vi "User Interface.vi"() -> ()   [LabVIEW 2015]
uses:
  <vilib>/Utility/error.llb/DialogType.ctl
  <vilib>/Instr/_visa.llb/VISA Configure Serial Port (Instr).vi
panel:
  out "Delta Psi 2":dbl
  out "Delta Psi":dbl
  out "Initial Stab":bool
  out "Initial Run":u32=1
  out "Automatic Mode Runtime":dbl
  out "ERROR":bool
  out "Theta i":dbl=177.58087201125176
  out "Psi i":dbl=181.08649789029536
  out "T initial read":u32
  out "Wzp":dbl(graph)
  out "Wyp":dbl(graph)=-0.09923664122137404
  out "Wxp":dbl(graph)=0.061068702290076333
  in  "Cluster":T1
  in  "Numeric":dbl=1.0
  out "return count":u32
  in  "Data Buffer":u8[](array[numeric])=[0, 8, 255, 243, 0, 0, 49, 1, 35, 1, 64, 0, 240, 0, 0, 3, 59, 255, 246, 0, 12, 0, 0, 48, 2, 35, 1, 64, 0, 240, 0, 0, 3, 27, 0, 0, 255, 244, 0, 0, 49, 1, 35, 1, 64, 0, 240, 0, 0, 2, 255, 0, 0, 255, 242, 0, 0, 49, 2, 35, 1, 64, 0, 240, 0, 0, 2, 225, 0, 9, 0, 0, 0, 0, 49, 1, 35, 1, 64, 0, 240, 0, 0, 2, 195, 0, 0, 0, 0, 0, 0, 48, 1, 35, 1, 64, 0, 240, 0, 0, 2, 167, 0, 0, 255, 248, 0, 0, 49, 1, 35, 1, 64, 0, 240, 0, 0, 2, 137, 0, 10, 0, 0, 0, 0, 49, 1, 35, 1, 64, 0, 240, 0, 0, 2, 109, 0, 0, 0, 0, 0, 0, 49, 1, 35, 1, 64, 0, 240, 0, 0, 2, 79, 0, 0, 0, 0, 0, 0, 49, 2, 35, 1, 64, 0, 240, 0, 0, 2, 49, 0, 0, 0, 0, 0, 0, 49, 1, 35, 1, 64, 0, 240, 0, 0, 2, 19, 0, 13, 255, 248, 0, 7, 49, 2, 35, 1, 64, 0, 240, 0, 0, 1, 247, 0, 0, 0, 12, 255, 245, 49, 1, 35, 1, 64, 0, 240, 0, 0, 1, 217, 0, 0, 0, 0, 0, 0, 49, 1, 35, 1, 64, 0, 240, 0, 0, 1, 189, 0, 0, 0, 12, 0, 0, 49, 1, 35, 1, 64, 0, 240, 0, 0, 1, 161, 0, 0, 255, 248, 0, 0, 49, 2, 35, 1, 64, 0, 240, 0, 0, 1, 131, 255, 249, 0, 0, 0, 9, 49, 2, 35, 1, 64, 0, 240, 0, 0, 1, 103, 0, 0, 255, 248, 0, 0, 49, 1, 35, 1, 64, 0, 240, 0, 0, 1, 74, 0, 0, 0, 0, 0, 0, 49, 1, 35, 1, 64, 0, 240, 0, 0, 1, 43, 0, 0, 0, 9, 0, 0, 49, 2, 35, 1, 64, 0, 240, 0, 0, 1, 13, 0, 0, 0, 7, 0, 0, 49, 2, 35, 1, 64, 0, 240, 0, 0, 0, 241, 0, 0, 0, 0, 0, 0, 49, 1, 35, 1, 64, 0, 240, 0, 0, 0, 211, 0, 0, 0, 0, 0, 0, 48, 2, 35, 1, 64, 0, 240, 0, 0, 0, 181, 0, 0, 0, 0, 0, 0, 49, 2, 35, 1, 64, 0, 240, 0, 0, 0, 151, 0, 0, 0, 0, 0, 0, 49, 1, 35, 1, 64, 0, 240, 0, 0, 0, 121, 0, 8, 0, 10, 0, 0, 48, 1, 35, 1, 64, 0, 240, 0, 0, 0, 91, 0, 0, 0, 0, 0, 0, 48, 2, 35, 1, 64, 0, 240, 0, 0, 0, 67, 0, 0, 0, 8, 0, 9, 48, 2, 35, 1, 64, 0, 240, 0, 0, 0, 63, 0, 0, 0, 0, 255, 243, 49, 2, 35, 1, 64, 0, 240, 0, 0, 0, 37, 0, 0, 0, 7, 0, 0, 49, 1, 35, 1, 64, 0, 240, 0, 0, 0, 5, 0, 0, 0, 0, 0, 0, 49, 2, 35, 1, 64, 0, 240, 0, 0, 0, 0]
  out "Psi":i16
  out "Theta":i16
  out "Cx":dbl=320.0
  out "Cy":dbl=240.0
  in  "Parity (0:none)":enum16{"None", "Odd", "Even", "Mark", "Space"}(ring)=enum."Even"
  in  "Phi B":dbl(slide) step=1.0 scale=-180.0..180.0
  in  "Psi B":dbl(slide) step=1.0 scale=-180.0..180.0
  in  "Theta B":dbl(slide) step=1.0 scale=-180.0..180.0
  in  "Tab Control":enum32{"MANUAL MODE", "AUTOMATIC MODE"}(tab)
  in  "Acquire \nTarget \nButton":bool
  in  "Yaw Angle":dbl(knob) caption="Pitch Angle" min=-90.0 max=90.0 step=1.0 scale=-90.0..90.0
  in  "Pitch Angle":dbl(knob) min=0.0 max=180.0 step=1.0
  in  "Start/Stop \nTracking":bool
  out "Target Position":dbl[][](graph)
  out "3D Picture":refnum<vi>(3d-picture)
  in  "stop":bool
  in  "VISA resource name":refnum<visa-resource-name>="COM4"
  in  "Stop bits (1 bit)":u16(ring)=10 items=["1.0"=10, "1.5"=15, "2.0"=20]
  in  "Baud rate":u32=115200
  # "SYSTEM SIMULATION"
  # "SERIAL COMMS SETUP"
  # "BASE MOTION"
  # "INERTIAL LOS RATES"
  # "SYSTEM STOP"
  # "SYSTEM COMMANDS"
  # "TARGET POSITION"
  # "Pitch Target"
  # "Yaw Target"
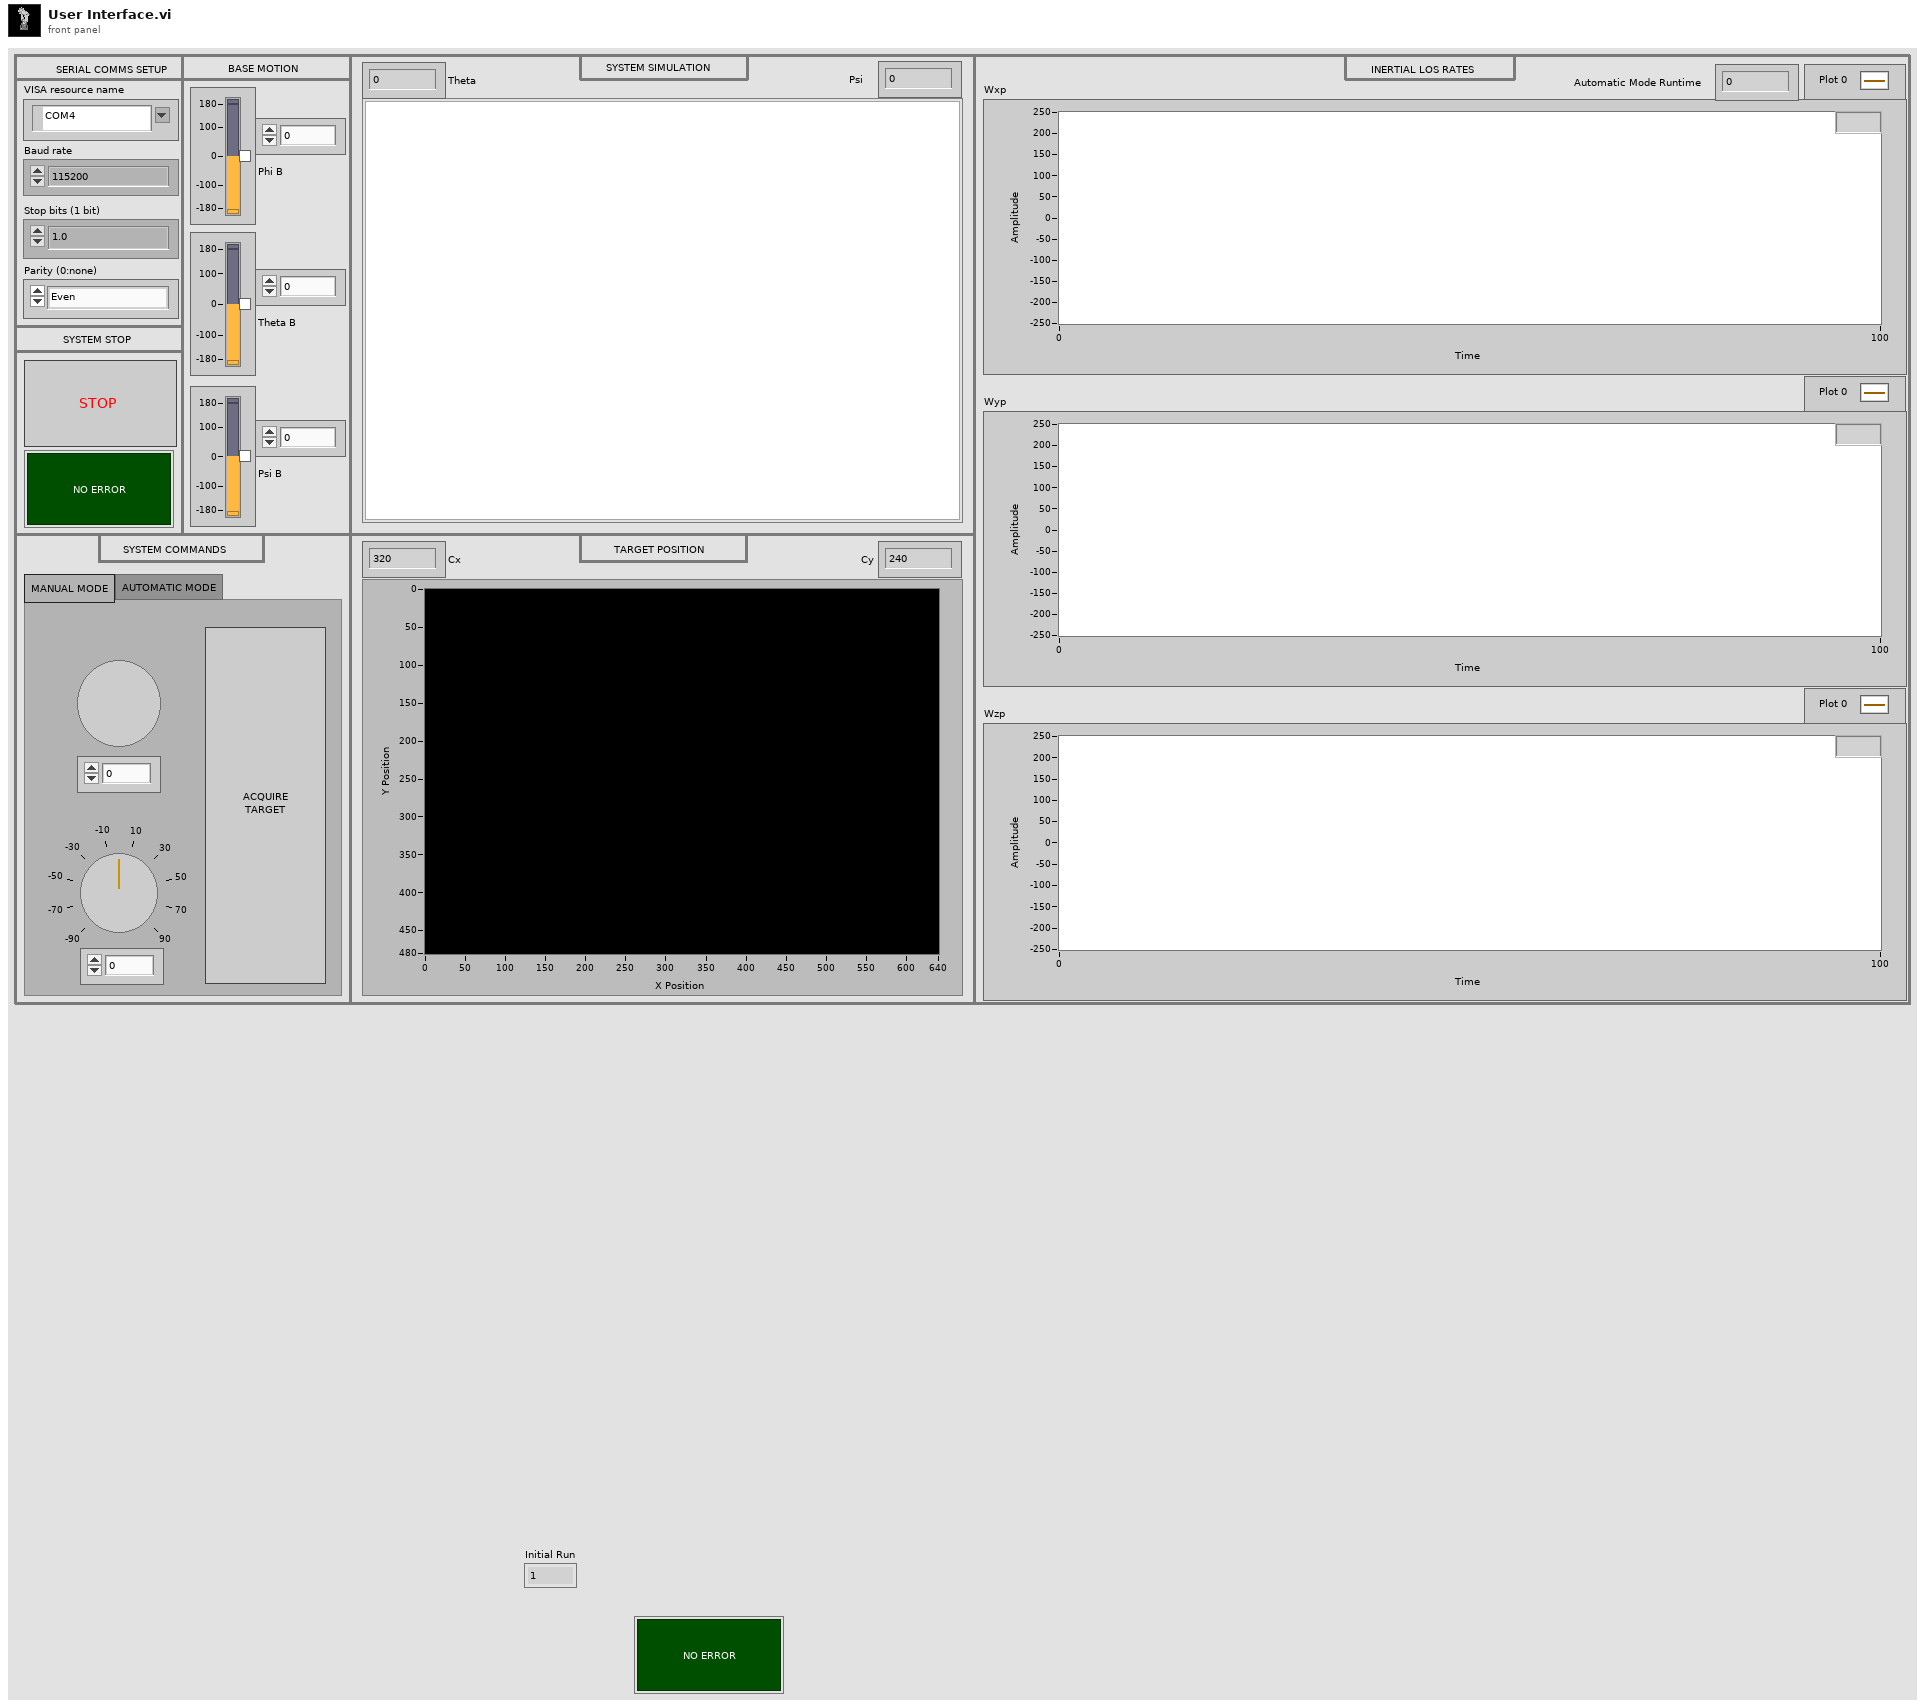
[diagram p1: front panel]
types:
  T1 = cluster{"X":dbl[], "Y":dbl[], "Z":dbl[], "theta":u16[], "phi":u16[], "CX":u16[], "CY":u16[], "Time":dbl[]}
  T2 = cluster{"Scene Object":refnum<vi>, "Base":refnum<vi>, "Gimbal":refnum<vi>, "Telescope":refnum<vi>, "error out":errorcluster}
  T3 = cluster{dbl[], dbl[], dbl[], u16[], u16[], u16[], u16[], dbl[]}
  T4 = typedef "DialogType.ctl" = u16
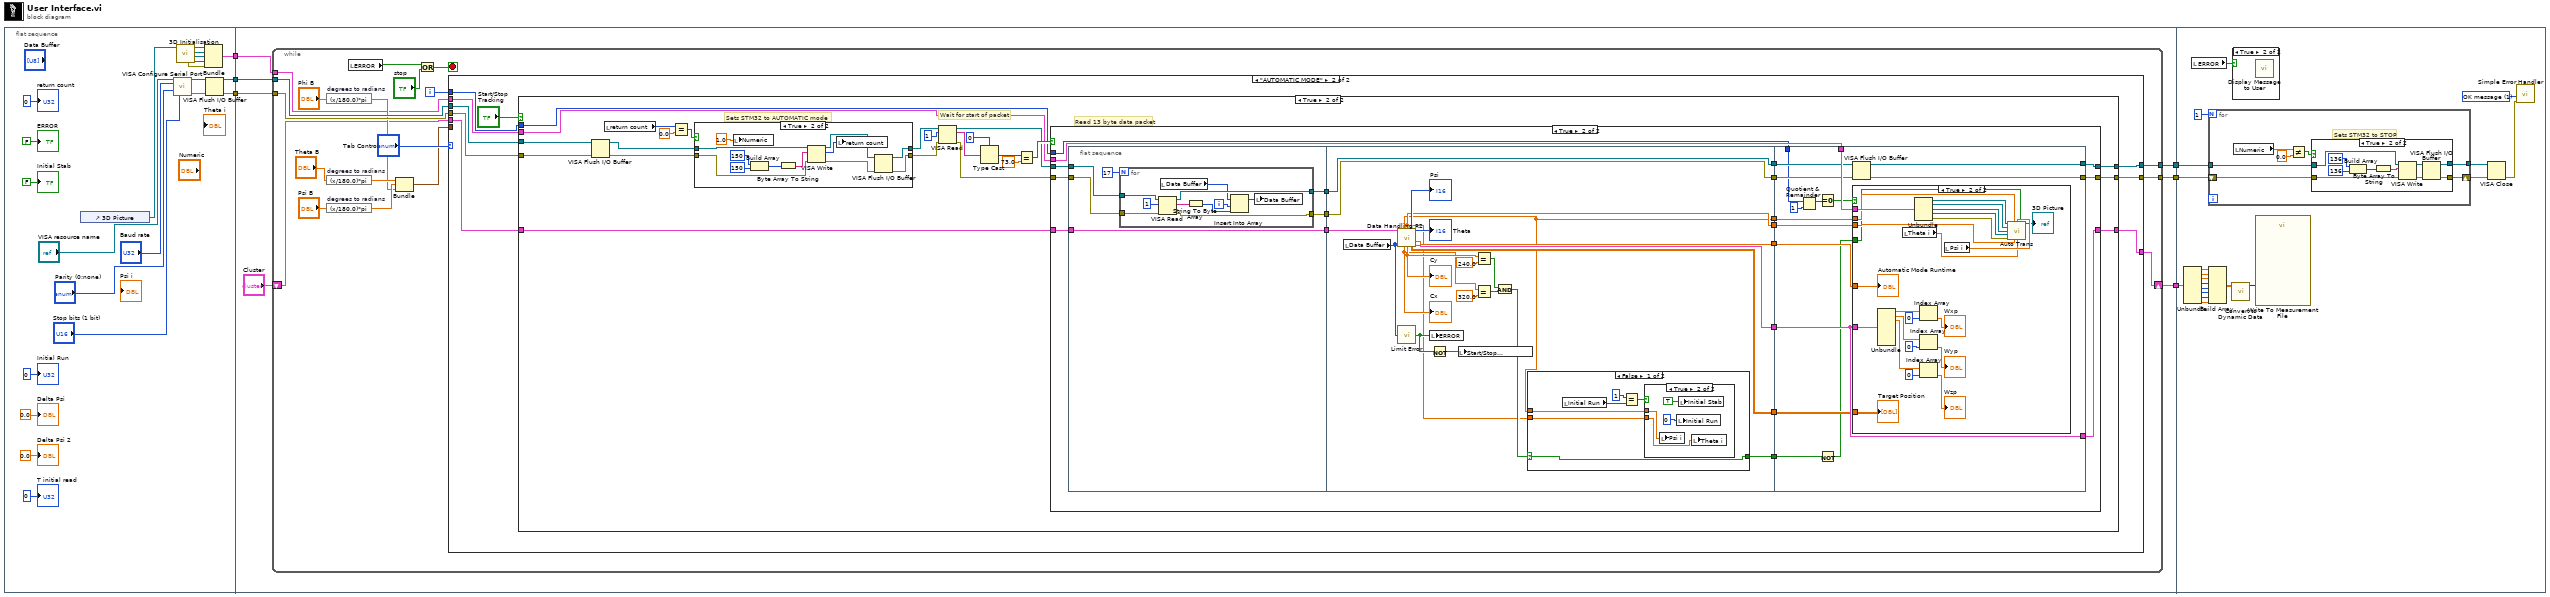
[diagram p0: block diagram]
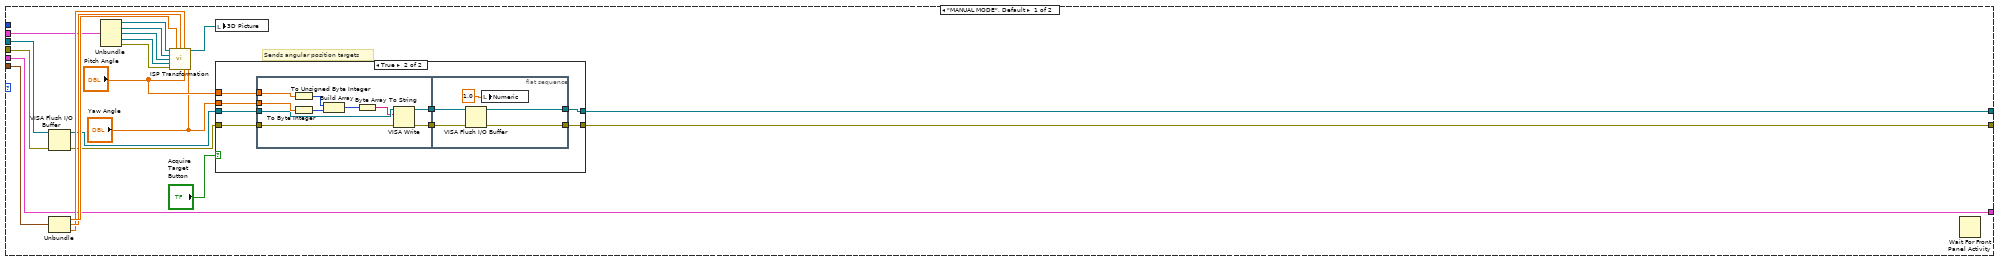
[diagram p2: hidden frame]
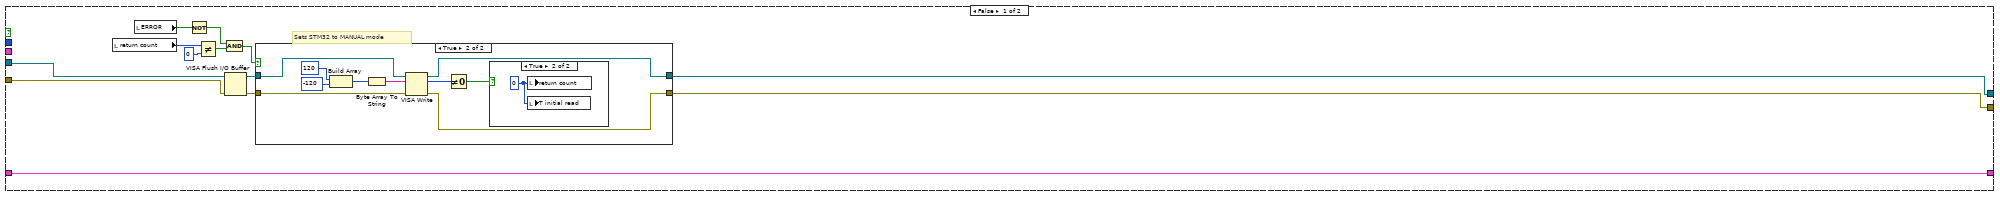
[diagram p4: hidden frame]
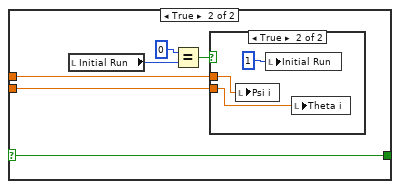
[diagram p9: hidden frame]
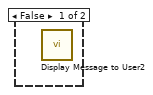
[diagram p14: hidden frame]
diagram:
  n1 = flat-sequence {
    tunnel: [w20] -> w6
    tunnel: [w19] -> w5
    tunnel: [w13] -> w4
    tunnel: w6 -> [w35]
    tunnel: w5 -> [w34]
    tunnel: w4 -> [w29]
    tunnel: [w32] -> w3
    tunnel: [w31] -> w2
    tunnel: [w30] -> w1
    tunnel: w3 -> [w308]
    tunnel: w2 -> [w307]
    tunnel: w1 -> [w306]
    frame #0 {
      n2 = control-ref of="3D Picture"() -> (w23:refnum<vi>)
      n3 = call-poly "VISA Configure Serial Port"("VISA resource name"="VISA resource name", "baud rate (9600)"="Baud rate", "parity (0:none)"="Parity (0:none)", "stop bits (10: 1 bit)"="Stop bits (1 bit)") -> ("VISA resource name out"=w22:refnum<visa-resource-name>, "error out"=w21:errorcluster)  [unwired: 10 in]
      n4 = call "3D Initialisation.vi"("reference"=w23) -> ("Telescope"=w15:refnum<vi>, "Gimbal"=w16:refnum<vi>, "Base"=w17:refnum<vi>, "Scene Object"=w18:refnum<vi>, "error out"=w14:errorcluster)  [unwired: 6 in]
      n5 = Bundle("Scene Object"=w18, "Base"=w17, "Gimbal"=w16, "Telescope"=w15, "error out"=w14) -> (w13:T2)  [unwired: 1 in]
      n6 = VISA Flush I/O Buffer(VISA resource name=w22, error in (no error)=w21) -> (VISA resource name out=w20:refnum<visa-resource-name>, error out=w19:errorcluster)  [unwired: 1 in]
      "return count" <- u32 0 ("return count")
      "T initial read" <- u32 0 ("initial read")
      "ERROR" <- FALSE ("LIMIT ERROR")
      "Initial Run" <- u32 0 ("initial read")
      "Initial Stab" <- FALSE ("LIMIT ERROR")
      "Delta Psi" <- 0.0 ("Delta Psi")
      "Delta Psi 2" <- 0.0 ("Delta Psi 2")
    }
    frame #1 {
      n7 = while {
        tunnel: w35 -> [w50]
        tunnel: w34 -> [w49]
        tunnel: w29 -> [w45]
        shift-right: [w43] -> w30
        shift-left: "Cluster" -> [w44]
        tunnel: [w42] -> w32
        tunnel: [w41] -> w31
        i -> [w36]
        stop <- w39 stop-if-true
        n8 = expression code="(x/180.0)*pi" "degrees to radians"("Phi B") -> (w46:dbl)
        n9 = expression code="(x/180.0)*pi" "degrees to radians"("Theta B") -> (w48:dbl)
        n10 = expression code="(x/180.0)*pi" "degrees to radians"("Psi B") -> (w47:dbl)
        n11 = local read "ERROR"() -> (w37:bool)
        n12 = Bundle("Theta B"=w48, "Psi B"=w47, "Phi B"=w46) -> (w40:cluster{"Theta B":dbl, "Psi B":dbl, "Phi B":dbl})  [unwired: 1 in]
        n13 = Or(x=w37, y="stop") -> (x .or. y?=w39:bool)
        n14 = case shown="\"AUTOMATIC MODE\"" "Tab Control" {
          tunnel: w50 -> [w56 w108]
          tunnel: w49 -> [w58 w107]
          tunnel: w44 -> [w63 w106]
          tunnel: w40 -> [w61 _]
          tunnel: w45 -> [w62 w105]
          tunnel: [w63 w104] -> w43
          tunnel: [w64 w103] -> w42
          tunnel: [w65 w102] -> w41
          tunnel: w36 -> [_ w101]
          frame "MANUAL MODE", Default {
            # "Sends angular position targets"
            n15 = VISA Flush I/O Buffer(VISA resource name=w56, error in (no error)=w58) -> (VISA resource name out=w55:refnum<visa-resource-name>, error out=w57:errorcluster)  [unwired: 1 in]
            n16 = Unbundle(w61) -> ("Theta B"=w70:dbl, "Psi B"=w69:dbl, "Phi B"=w68:dbl)
            n17 = Unbundle(w62) -> ("Scene Object"=w75:refnum<vi>, "Base"=w74:refnum<vi>, "Gimbal"=w73:refnum<vi>, "Telescope"=w72:refnum<vi>, "error out"=w71:errorcluster)
            n18 = call "ISP Transformation.vi"("Scene Object In"=w75, "Theta B"=w70, "Psi B"=w69, "Phi B"=w68, "Base"=w74, "Gimbal"=w73, "Telescope"=w72, "error in (no error)"=w71, "Theta"="Pitch Angle", "Psi"="Yaw Angle") -> ("Scene Object Out"=w67:refnum<vi>)  [unwired: 4 in, 1 out]
            n19 = local write "3D Picture"(w67) -> ()
            n20 = case shown="True" "Acquire \nTarget \nButton" {
              tunnel: "Pitch Angle" -> [_ w85]
              tunnel: "Yaw Angle" -> [_ w84]
              tunnel: w55 -> [w77 w83]
              tunnel: w57 -> [w76 w82]
              tunnel: [w76 w78] -> w65
              tunnel: [w77 w79] -> w64
              frame False {
              }
              frame True {
                n21 = flat-sequence {
                  tunnel: w85 -> [w95]
                  tunnel: w84 -> [w94]
                  tunnel: w83 -> [w93]
                  tunnel: w82 -> [w92]
                  tunnel: [w91] -> w81
                  tunnel: [w90] -> w80
                  tunnel: [w98] -> w78
                  tunnel: [w97] -> w79
                  tunnel: w81 -> [w96]
                  tunnel: w80 -> [w99]
                  frame #0 {
                    n22 = To Unsigned Byte Integer(number=w95) -> (unsigned 8bit integer=w87:u8)
                    n23 = To Byte Integer(number=w94) -> (8bit integer=w88:i8)
                    n24 = Build Array(w87, w88) -> (w89:u8[])
                    n25 = Byte Array To String(unsigned byte array=w89) -> (string=w86:string)
                    n26 = VISA Write(VISA resource name=w93, write buffer=w86, error in (no error)=w92) -> (VISA resource name out=w91:refnum<visa-resource-name>, error out=w90:errorcluster)  [unwired: 1 out]
                  }
                  frame #1 {
                    n27 = VISA Flush I/O Buffer(VISA resource name=w96, error in (no error)=w99) -> (VISA resource name out=w97:refnum<visa-resource-name>, error out=w98:errorcluster)  [unwired: 1 in]
                    n28 = local write "Numeric"(1.0 ("Numeric")) -> ()
                  }
                }
              }
            }
            n29 = Wait For Front Panel Activity() -> ()  [unwired: 3 in, 1 out]
          }
          frame "AUTOMATIC MODE" {
            n30 = case shown="True" "Start/Stop \nTracking" {
              tunnel: w108 -> [w113 w137]
              tunnel: w107 -> [w110 w136]
              tunnel: w106 -> [w118 w145]
              tunnel: w105 -> [_ w144]
              tunnel: [w118 w143] -> w104
              tunnel: [w120 w142] -> w103
              tunnel: [w119 w141] -> w102
              tunnel: w101 -> [_ w140]
              frame False {
                # "Sets STM32 to MANUAL mode"
                n31 = local read "return count"() -> (w121:u32)
                n32 = local read "ERROR"() -> (w115:bool)
                n33 = Not(x=w115) -> (.not. x?=w114:bool)
                n34 = Not Equal?(x=w121, y=u32 0) -> (x != y?=w116:bool)
                n35 = And(x=w114, y=w116) -> (x .and. y?=w117:bool)
                n36 = VISA Flush I/O Buffer(VISA resource name=w113, error in (no error)=w110) -> (VISA resource name out=w112:refnum<visa-resource-name>, error out=w111:errorcluster)  [unwired: 1 in]
                n37 = case shown="True" w117 {
                  tunnel: w112 -> [w124 w134]
                  tunnel: w111 -> [w123 w133]
                  tunnel: [w124 w132] -> w120
                  tunnel: [w123 w131] -> w119
                  frame False {
                  }
                  frame True {
                    n38 = Build Array(i8 120 ("element"), i8 -120 ("element")) -> (w127:i8[])
                    n39 = Byte Array To String(unsigned byte array=w127) -> (string=w130:string)
                    n40 = VISA Write(VISA resource name=w134, write buffer=w130, error in (no error)=w133) -> (VISA resource name out=w132:refnum<visa-resource-name>, return count=w125:u32, error out=w131:errorcluster)
                    n41 = Not Equal To 0?(x=w125) -> (x != 0?=w126:bool)
                    n42 = case shown="True" w126 {
                      frame False {
                      }
                      frame True {
                        w135 = u32 0 ("return count")
                        n43 = local write "return count"(w135) -> ()
                        n44 = local write "T initial read"(w135) -> ()
                      }
                    }
                  }
                }
              }
              frame True {
                # "Wait for start of packet"
                # "Read 13 byte data packet"
                # "Sets STM32 to AUTOMATIC mode"
                n45 = VISA Flush I/O Buffer(VISA resource name=w137, error in (no error)=w136) -> (VISA resource name out=w139:refnum<visa-resource-name>, error out=w138:errorcluster)  [unwired: 1 in]
                n46 = local read "return count"() -> (w156:u32)
                n47 = Equal?(x=w156, y=0.0) -> (x = y?=w158:bool)
                n48 = case shown="True" w158 {
                  tunnel: w139 -> [w278 w286]
                  tunnel: w138 -> [w277 w285]
                  tunnel: [w278 w281] -> w154
                  tunnel: [w277 w280] -> w153
                  frame False {
                  }
                  frame True {
                    n49 = local write "Numeric"(1.0 ("Numeric")) -> ()
                    n50 = Build Array(u8 150 ("element"), u8 150 ("element")) -> (w287:u8[])
                    n51 = Byte Array To String(unsigned byte array=w287) -> (string=w290:string)
                    n52 = VISA Write(VISA resource name=w286, write buffer=w290, error in (no error)=w285) -> (VISA resource name out=w284:refnum<visa-resource-name>, return count=w282:u32, error out=w283:errorcluster)
                    n53 = local write "return count"(w282) -> ()
                    n54 = VISA Flush I/O Buffer(VISA resource name=w284, error in (no error)=w283) -> (VISA resource name out=w281:refnum<visa-resource-name>, error out=w280:errorcluster)  [unwired: 1 in]
                  }
                }
                n55 = VISA Read(VISA resource name=w154, byte count=u32 1, error in (no error)=w153) -> (VISA resource name out=w147:refnum<visa-resource-name>, read buffer=w149:string, error out=w146:errorcluster)  [unwired: 1 out]
                n56 = Type Cast(type=u8 0, x=w149) -> (*(type *) &x=w151:u8)
                n57 = Equal?(x=w151, y=73.0) -> (x = y?=w148:bool)
                n58 = case shown="True" w148 {
                  tunnel: w147 -> [w160 w175]
                  tunnel: w146 -> [w159 w174]
                  tunnel: w145 -> [w161 w176]
                  tunnel: w144 -> [_ w180]
                  tunnel: [w161 w169] -> w143
                  tunnel: [w160 w179] -> w142
                  tunnel: [w159 w178] -> w141
                  tunnel: w140 -> [_ w177]
                  frame False {
                  }
                  frame True {
                    n59 = flat-sequence {
                      tunnel: w174 -> [w181]
                      tunnel: w175 -> [w182]
                      tunnel: [w185] -> w173
                      tunnel: [w184] -> w172
                      tunnel: w176 -> [w185]
                      tunnel: [w183] -> w171
                      tunnel: w173 -> [w207]
                      tunnel: w172 -> [w200]
                      tunnel: w171 -> [w201]
                      tunnel: [w201] -> w170
                      tunnel: [w206] -> w168
                      tunnel: [w205] -> w167
                      tunnel: [w204] -> w166
                      tunnel: [w203] -> w165
                      tunnel: [w202] -> w164
                      tunnel: [w200] -> w163
                      tunnel: [w199] -> w162
                      tunnel: [w243] -> w169
                      tunnel: w180 -> [w252]
                      tunnel: [w251] -> w179
                      tunnel: [w248] -> w178
                      tunnel: w177 -> [w247]
                      tunnel: w170 -> [w250]
                      tunnel: w168 -> [w243]
                      tunnel: w167 -> [w242]
                      tunnel: w166 -> [w241]
                      tunnel: w165 -> [w240]
                      tunnel: w164 -> [w239]
                      tunnel: w163 -> [w249]
                      tunnel: w162 -> [w238]
                      frame #0 {
                        n60 = for {
                          N: 17 -> [_]
                          tunnel: [w195] -> w183
                          tunnel: [w194] -> w184
                          tunnel: w182 -> [w188]
                          tunnel: w181 -> [w187]
                          i -> [w189]
                          n61 = VISA Read(VISA resource name=w188, byte count=u32 1, error in (no error)=w187) -> (VISA resource name out=w195:refnum<visa-resource-name>, read buffer=w193:string, error out=w194:errorcluster)  [unwired: 1 out]
                          n62 = local read "Data Buffer"() -> (w191:u8[])
                          n63 = String To Byte Array(string=w193) -> (unsigned byte array=w192:u8[])
                          n64 = Insert Into Array(array=w191, index=w189, new element=w192) -> (w190:u8[])
                          n65 = local write "Data Buffer"(w190) -> ()
                        }
                      }
                      frame #1 {
                        n66 = local read "Data Buffer"() -> (w208:u8[])
                        n67 = call "Data Handling R2.vi"("Cluster"=w207, "Data Buffer"=w208) -> ("Psi (image)"=w202:dbl, "Theta (image)"=w203:dbl, "Psi array out"=→"Psi":i16, "Theta array out"=→"Theta":i16, "Time"=w205:dbl, "Cx"=w213:dbl, "Cy"=w214:dbl, "Target array"=w204:dbl[][], "output cluster"=w206:T3)  [unwired: 5 in]
                        "Cy" <- w214
                        "Cx" <- w213
                        n68 = call "Limit Error.vi"("Array"=w208) -> ("LIMIT ERROR"=w210:bool)
                        n69 = local write "ERROR"(w210) -> ()
                        n70 = Not(x=w210) -> (.not. x?=w209:bool)
                        n71 = local write "Start/Stop \nTracking"(w209) -> ()
                        n72 = Equal?(x=w214, y=240.0) -> (x = y?=w198:bool)
                        n73 = Equal?(x=w213, y=320.0) -> (x = y?=w197:bool)
                        n74 = And(x=w198, y=w197) -> (x .and. y?=w215:bool)
                        n75 = case shown="False" w215 {
                          selector: w215 -> [w218 w228]
                          tunnel: w202 -> [w220 w230]
                          tunnel: w203 -> [w219 w229]
                          tunnel: [w218 w228] -> w199
                          frame False {
                            n76 = local read "Initial Run"() -> (w222:u32)
                            n77 = Equal?(x=u32 1, y=w222) -> (x = y?=w221:bool)
                            n78 = case shown="True" w221 {
                              tunnel: w220 -> [_ w226]
                              tunnel: w219 -> [_ w225]
                              frame False {
                              }
                              frame True {
                                n79 = local write "Psi i"(w226) -> ()
                                n80 = local write "Initial Run"(u32 0 ("T initial read")) -> ()
                                n81 = local write "Initial Stab"(TRUE ("Initial Stab")) -> ()
                                n82 = local write "Theta i"(w225) -> ()
                              }
                            }
                          }
                          frame True {
                            n83 = local read "Initial Run"() -> (w232:u32)
                            n84 = Equal?(x=u32 0, y=w232) -> (x = y?=w231:bool)
                            n85 = case shown="True" w231 {
                              tunnel: w230 -> [_ w236]
                              tunnel: w229 -> [_ w235]
                              frame False {
                              }
                              frame True {
                                n86 = local write "Psi i"(w236) -> ()
                                n87 = local write "Initial Run"(u32 1 ("initial read")) -> ()
                                n88 = local write "Theta i"(w235) -> ()
                              }
                            }
                          }
                        }
                      }
                      frame #2 {
                        n89 = Quotient & Remainder(x=w247, y=1) -> (x-y*floor(x/y)=w245:i32)  [unwired: 1 out]
                        n90 = Equal To 0?(x=w245) -> (x = 0?=w244:bool)
                        n91 = Not(x=w238) -> (.not. x?=w237:bool)
                        n92 = VISA Flush I/O Buffer(VISA resource name=w250, error in (no error)=w249) -> (VISA resource name out=w251:refnum<visa-resource-name>, error out=w248:errorcluster)  [unwired: 1 in]
                        n93 = case shown="True" w244 {
                          tunnel: w252 -> [_ w273]
                          tunnel: w243 -> [_ w272]
                          tunnel: w241 -> [_ w265]
                          tunnel: w240 -> [_ w261]
                          tunnel: w239 -> [_ w255]
                          tunnel: w242 -> [_ w264]
                          tunnel: w237 -> [_ w253]
                          frame False {
                          }
                          frame True {
                            n94 = Unbundle(w272) -> (w271:dbl[], w270:dbl[], w269:dbl[])  [unwired: 5 out]
                            n95 = local read "Theta i"() -> (w262:dbl)
                            n96 = Unbundle(w273) -> ("Scene Object"=w256:refnum<vi>, "Base"=w257:refnum<vi>, "Gimbal"=w258:refnum<vi>, "Telescope"=w259:refnum<vi>, "error out"=w260:errorcluster)
                            n97 = Index Array(array=w271, index=0) -> (element=→"Wxp":dbl)
                            n98 = Index Array(array=w270, index=0) -> (element=→"Wyp":dbl)
                            n99 = Index Array(array=w269, index=0) -> (element=→"Wzp":dbl)
                            n100 = local read "Psi i"() -> (w263:dbl)
                            n101 = call "Auto Trans.vi"("Scene Object In"=w256, "Psi"=w255, "Psi i"=w263, "Boolean"=w253, "Base"=w257, "Gimbal"=w258, "Telescope"=w259, "error in (no error)"=w260, "Theta"=w261, "Theta i"=w262) -> ("Scene Object Out"=→"3D Picture":refnum<vi>)  [unwired: 4 in, 1 out]
                            "Target Position" <- w265
                            "Automatic Mode Runtime" <- w264
                          }
                        }
                      }
                    }
                  }
                }
              }
            }
          }
        }
      }
    }
    frame #2 {
      w309 = T4 1 items=["no dialog", "OK message", "continue or stop message", "OK message + warnings", "continue/stop + warnings"] ("type of dialog (OK msg:1)")
      n102 = Unbundle(w306) -> ("X"=w305:dbl[], "Y"=w304:dbl[], "Z"=w303:dbl[], "theta"=w302:u16[], "phi"=w301:u16[], "CX"=w300:u16[], "CY"=w299:u16[], "Time"=w294:dbl[])
      n103 = local read "ERROR"() -> (w296:bool)
      n104 = for {
        N: 1 -> [_]
        tunnel: w308 -> [w314]
        shift-right: [w311] -> w293
        shift-left: w307 -> [w313]
        tunnel: [w310] -> w291
        # "Sets STM32 to STOP"
        n105 = local read "Numeric"() -> (w312:dbl)
        n106 = Not Equal?(x=w312, y=0.0) -> (x != y?=w315:bool)
        n107 = case shown="True" w315 {
          tunnel: [w318 w320] -> w311
          tunnel: w314 -> [w317 w324]
          tunnel: w313 -> [w318 w323]
          tunnel: [w317 w319] -> w310
          frame False {
          }
          frame True {
            n108 = Build Array(u8 136 ("element"), u8 136 ("element")) -> (w325:u8[])
            n109 = Byte Array To String(unsigned byte array=w325) -> (string=w328:string)
            n110 = VISA Write(VISA resource name=w324, write buffer=w328, error in (no error)=w323) -> (VISA resource name out=w322:refnum<visa-resource-name>, error out=w321:errorcluster)  [unwired: 1 out]
            n111 = VISA Flush I/O Buffer(VISA resource name=w322, error in (no error)=w321) -> (VISA resource name out=w319:refnum<visa-resource-name>, error out=w320:errorcluster)  [unwired: 1 in]
          }
        }
      }
      n112 = Build Array(w305, w304, w303, w302, w301, w300, w299, w294) -> (w298:dbl[][])
      n113 = call "Convert to Dynamic Data"("2D Array"=w298) -> ("Dynamic Data Type"=w297:dynamicdata)  [unwired: 3 in]
      n114 = case shown="True" w296 {
        frame False {
          n115 = call "Display Message to User2"() -> ()  [unwired: 10 in, 2 out]
        }
        frame True {
          n116 = call "Display Message to User"() -> ()  [unwired: 10 in, 2 out]
        }
      }
      n117 = call "Write To Measurement File"("Signals"=w297) -> ()  [unwired: 16 in, 3 out]
      n118 = VISA Close(VISA resource name=w291, error in (no error)=w293) -> (error out=w292:errorcluster)
      n119 = call <vilib>:"Simple Error Handler.vi"("type of dialog (OK msg:1)"=w309, "error in (no error)"=w292) -> ()  [unwired: 3 in, 5 out]
    }
  }
